vi "Autonomous Independent.vi"() -> ()   [LabVIEW 2017]
doc: "This VI is called when autonomous begins, and will automatically be terminated when autonomous ends. You can carry out timed or sensor driven robot movement independently without needing to return to the caller."
uses:
  Step Autonomous/TypeDefAuto.ctl
  Step Autonomous/TypeDefEnumSelection.ctl
  <vilib>/Rock Robotics/Network Tables/NT Read String.vi
  <vilib>/Rock Robotics/Network Tables/NT Write String.vi
  <vilib>/Rock Robotics/WPI/RobotDrive/WPI_RobotDriveArcadeDrive_Standard(NoSaturation).vi
  <vilib>/Rock Robotics/Network Tables/NT Write Numeric Array.vi
panel:
  out "directvi":string
  out "dashboard":string
  out "global":string
  out "Current Movement, for debugging":T1 {"Y Joystick Value" scale=1.0..-1.0; "X Joystick Value" scale=-1.0..1.0}
  in  "Array of robot movements":T2(array[cluster])=[{"X Joystick Value"=0.39393939393939403, "Y Joystick Value"=0.0, "Delay (sec)"=1.0, "Movement Name"="turn"}, {"X Joystick Value"=-0.3737373737373737, "Y Joystick Value"=0.0, "Delay (sec)"=1.0, "Movement Name"="turn back"}] {"Y Joystick Value" scale=1.0..-1.0; "X Joystick Value" scale=-1.0..1.0}
  # "Be sure to right-click and choose Data Operations>>Make Current Value default if you want to save the array values with the VI"
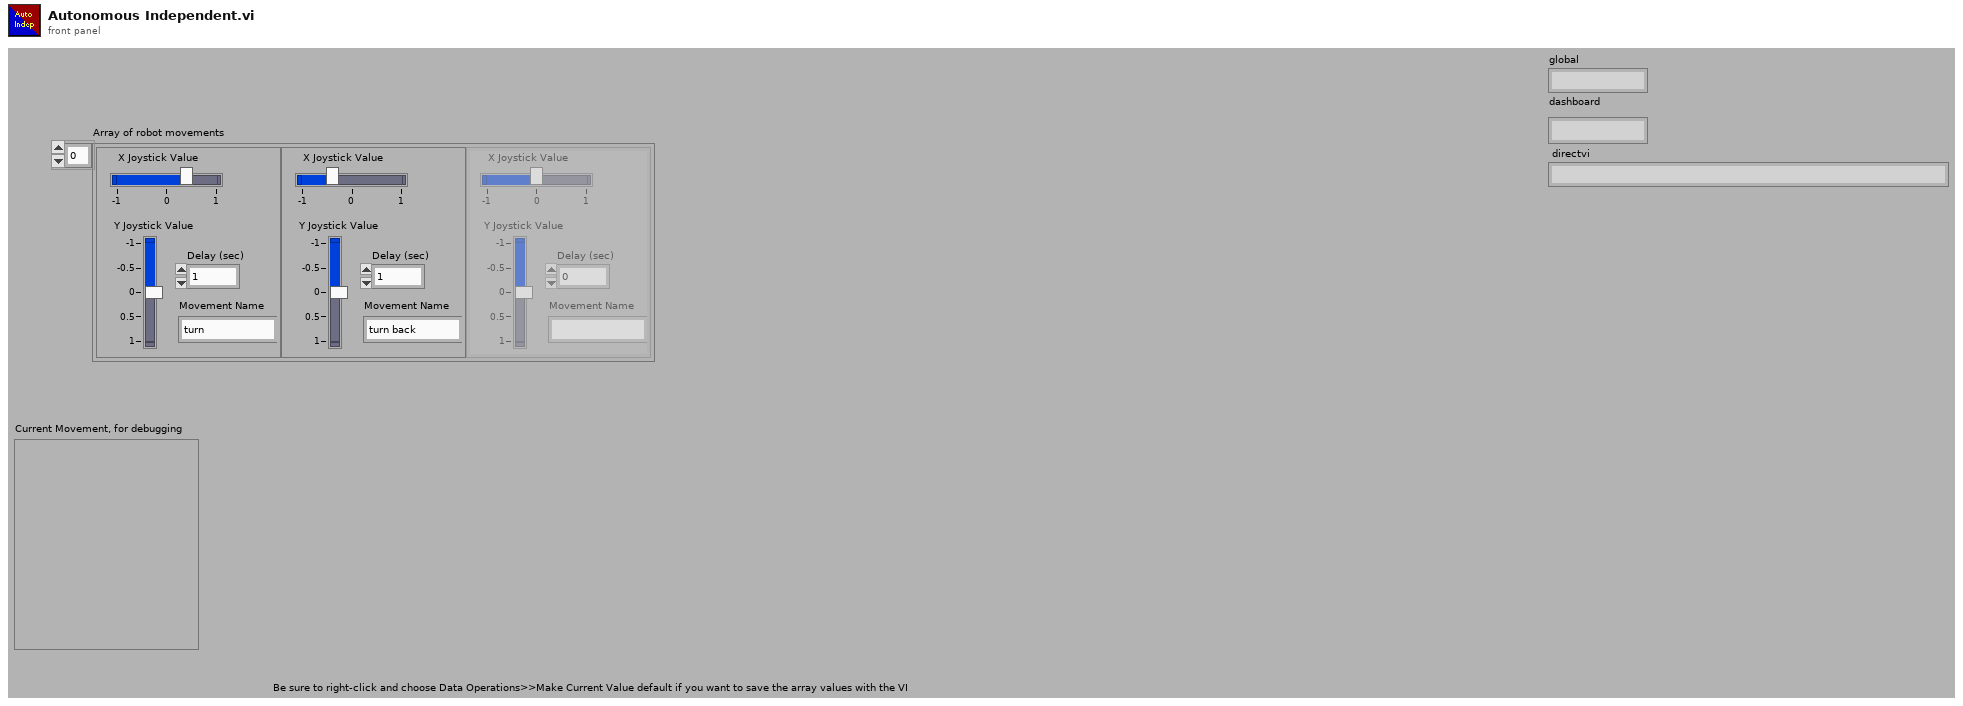
[diagram p1: front panel]
types:
  T1 = cluster{"X Joystick Value":dbl, "Y Joystick Value":dbl, "Delay (sec)":dbl, "Movement Name":string}
  T2 = cluster{"X Joystick Value":dbl, "Y Joystick Value":dbl, "Delay (sec)":dbl, "Movement Name":string}[]
  T3 = typedef "WPI_RobotDriveDevRef.ctl" = cluster{"DevStatus":errorcluster, "Motors[]":T4[], "Square Inputs":bool, "Max Output":dbl}
  T4 = typedef "WPI_MotorControlDeviceRef.ctl" = cluster{"DeviceStatus":errorcluster, "Type":T5, "PWM":cluster{"PWM Channel":T6, "DeadBand":T7}, "CAN":cluster{"Device Number":u8, "SetOutput VI Ref":variant, "GetOutput VI Ref":variant, "Enable VI Ref":variant, "Disable VI Ref":variant, "Data":variant}, "Invert":bool, "DIO PWM":cluster{"PWM \"Enable\" Channel":T6, "DIOChannel":T8, "PWM Rate":dbl}}
  T5 = typedef "WPI_MotorControlType.ctl" = enum16{"PWM", "CAN", "DIO PWM"}
  T6 = typedef "FPGA_DIOPWMChannel.ctl" = enum8{"PWM 0", "PWM 1", "PWM 2", "PWM 3", "PWM 4", "PWM 5", "PWM 6", "PWM 7", "PWM 8", "PWM 9", "PWM MXP 0", "PWM MXP 1", "PWM MXP 2", "PWM MXP 3", "PWM MXP 4", "PWM MXP 5", "PWM MXP 6", "PWM MXP 7", "PWM MXP 8", "PWM MXP 9", "Invalid"}
  T7 = typedef "WPI_PWMDeadband.ctl" = cluster{"Name":string, "maxPositivePwm":i32, "minPositivePwm":i32, "centerPwm":i32, "maxNegativePwm":i32, "minNegativePwm":i32, "angularRange":u16}
  T8 = typedef "FPGA_DIOChannel.ctl" = enum8{"DIO 0", "DIO 1", "DIO 2", "DIO 3", "DIO 4", "DIO 5", "DIO 6", "DIO 7", "DIO 8", "DIO 9", "DIO MXP 0", "DIO MXP 1", "DIO MXP 2", "DIO MXP 3", "DIO MXP 4", "DIO MXP 5", "DIO MXP 6", "DIO MXP 7", "DIO MXP 8", "DIO MXP 9", "DIO MXP 10", "DIO MXP 11", "DIO MXP 12", "DIO MXP 13", "DIO MXP 14", "DIO MXP 15", "SPI Port CS1", "SPI Port CS2", "SPI Port CS3", "SPI Port MISO", "SPI Port MOSI", "Invalid"}
  T9 = typedef "TypeDefAuto.ctl" = cluster{"Selection":T10, "Magnitude":dbl}
  T10 = typedef "TypeDefEnumSelection.ctl" = enum16{"Intake", "Drive", "Turn", "Lift", "Eject", "Wait", "RaiseDrop", "FastDrive", "VisionDrive", "TimedDrive"}
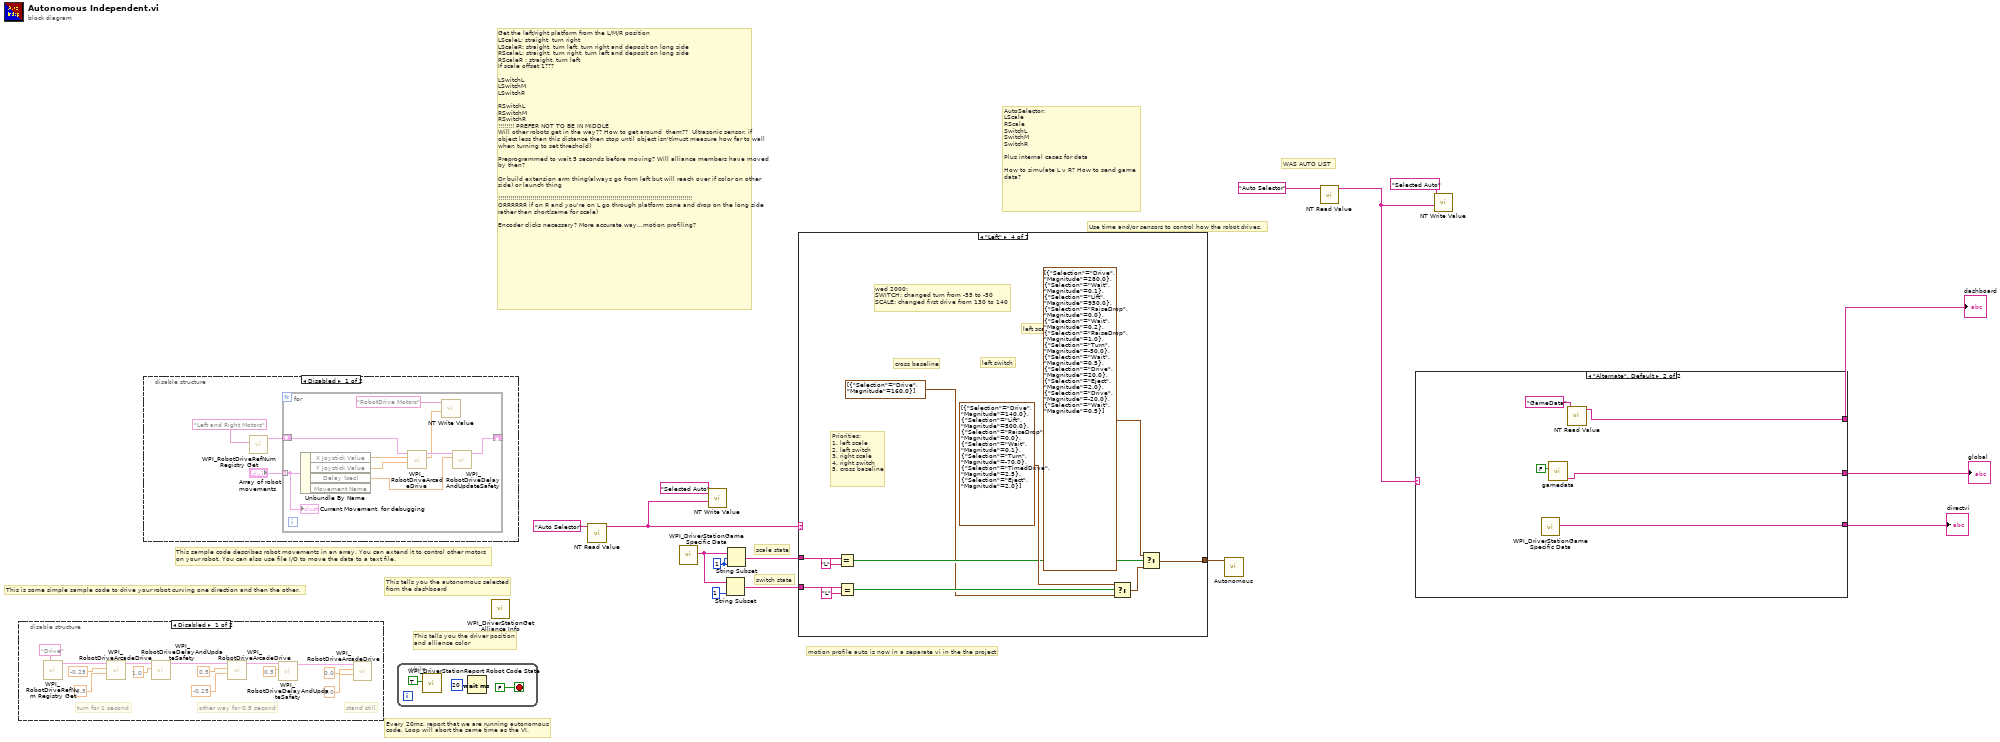
[diagram p0: block diagram]
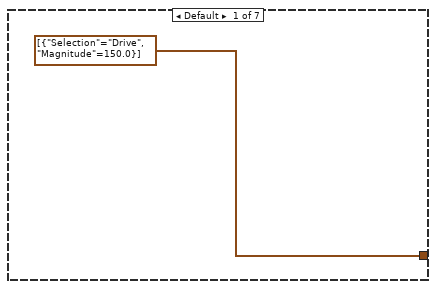
[diagram p2: hidden frame]
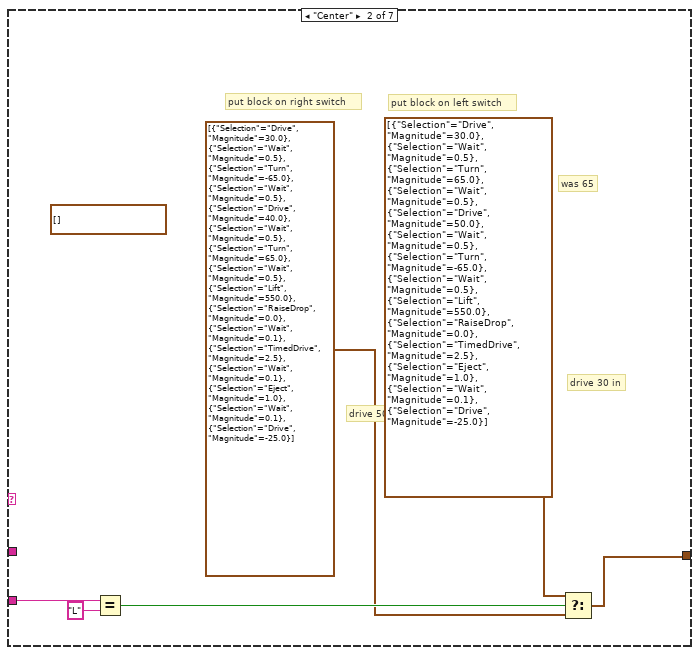
[diagram p3: hidden frame]
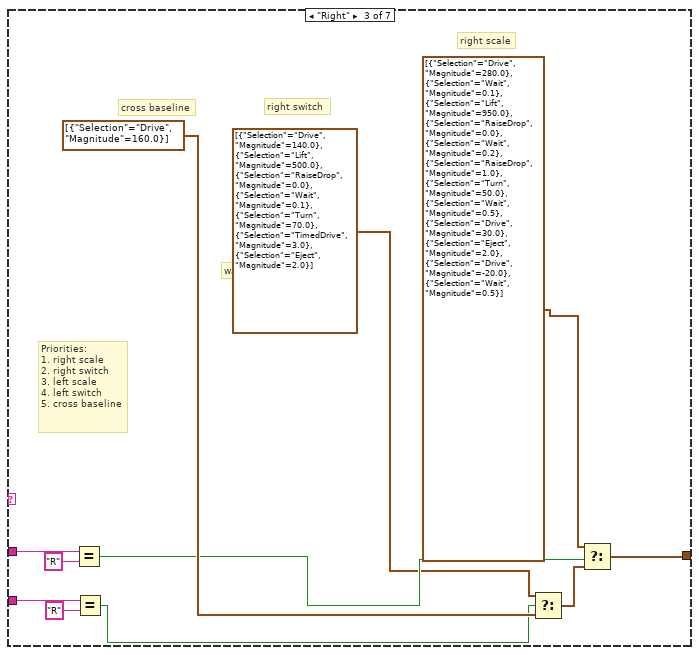
[diagram p4: hidden frame]
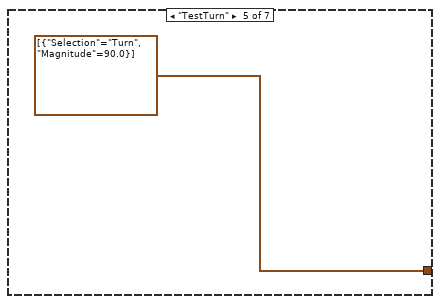
[diagram p5: hidden frame]
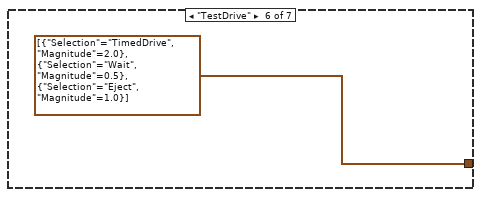
[diagram p6: hidden frame]
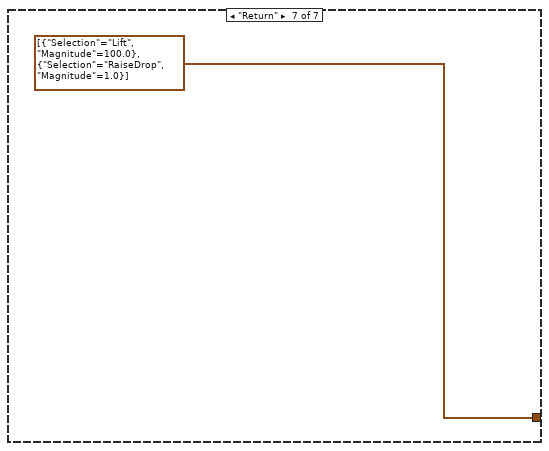
[diagram p7: hidden frame]
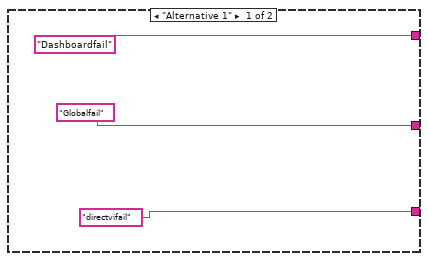
[diagram p8: hidden frame]
diagram:
  w2 = 1 ("length (rest)")
  # "motion profile auto is now in a separate vi in the the project"
  # "scale state"
  # "switch state"
  # "Use time and/or sensors to control how the robot drives."
  # "AutoSelector: \nLScale\nRScale\nSwitchL\nSwitchM\nSwitchR\n\nPlus internal cases for data\n\nHow to simulate L v R? How to send game data?"
  # "WAS AUTO LIST"
  # "This is some simple sample code to drive your robot curving one direction and then the other."
  # "This sample code describes robot movements in an array. You can extend it to control other motors\non your robot. You can also use file I/O to move the data to a text file."
  # "Get the left/right platform from the L/M/R position\nLScaleL: straight, turn right\nLScaleR: straight, turn left, turn right and deposit on long side\nRScaleL: straight, turn right, turn left and deposit on long side \nRScaleR : straight, turn left\nIf scale offset 1???\n\nLSwitchL\nLSwitchM\nLSwitchR\n\nRSwitchL\nRSwitchM\nRSwitchR\n!!!!!!!! PREFER NOT TO BE IN MIDDLE\nWill other robots get in the way?? How to get around  them??  Ultrasonic sensor, if object less than this distance then stop until object isn't(must measure how far to wall when turning to set threshold)\n\nPreprogrammed to wait 5 seconds before moving? Will alliance members have moved by then?\n\nOr build extension arm thing(always go from left but will reach over if color on other side) or launch thing\n\n!!!!!!!!!!!!!!!!!!!!!!!!!!!!!!!!!!!!!!!!!!!!!!!!!!!!!!!!!!!!!!!!!!!!!!!!!!!!!!!!!!!!!!!!!!!!!!!!!\nORRRRRR if on R and you're on L go through platform zone and drop on the long side rather than short(same for scale)  \n\nEncoder clicks necessary? More accurate way...motion profiling?"
  # "This tells you the autonomous selected\nfrom the dashboard"
  # "Every 20ms, report that we are running autonomous\ncode. Loop will abort the same time as the VI."
  # "This tells you the driver position\nand alliance color"
  n1 = disable-structure shown="Disabled" {
    frame Disabled {
      # "stand still"
      # "other way for 0.5 second"
      # "turn for 1 second"
      n2 = call <vilib>:"WPI_RobotDriveRefNum Registry Get.vi"("refnum name"="Drive") -> ("RobotDriveDevRef"=w25:T3)  [unwired: 1 in, 9 out]
      n3 = call-poly <vilib>:"WPI_RobotDriveArcadeDrive.vi"("Y axis value"=0.5 ("X axis value"), "X axis value"=-0.25, "RobotDriveDevRef"=w25) -> ("RobotDriveDevRef"=w29:T3)  [unwired: 1 in, 7 out]
      n4 = call <vilib>:"WPI_RobotDriveDelayAndUpdateSafety.vi"("Delay (s)"=1.0, "RobotDriveDevRef"=w29) -> ("RobotDriveDevRef 2"=w28:T3)  [unwired: 8 in, 1 out]
      n5 = call-poly <vilib>:"WPI_RobotDriveArcadeDrive.vi"("Y axis value"=-0.25 ("X axis value"), "X axis value"=0.5, "RobotDriveDevRef"=w28) -> ("RobotDriveDevRef"=w27:T3)  [unwired: 1 in, 7 out]
      n6 = call <vilib>:"WPI_RobotDriveDelayAndUpdateSafety.vi"("Delay (s)"=0.5, "RobotDriveDevRef"=w27) -> ("RobotDriveDevRef 2"=w26:T3)  [unwired: 8 in, 1 out]
      n7 = call-poly <vilib>:"WPI_RobotDriveArcadeDrive.vi"("Y axis value"=0.0 ("X axis value"), "X axis value"=0.0, "RobotDriveDevRef"=w26) -> ()  [unwired: 1 in, 8 out]
    }
    frame Enabled {
    }
  }
  n8 = disable-structure shown="Disabled" {
    frame Disabled {
      n9 = call <vilib>:"WPI_RobotDriveRefNum Registry Get.vi"("refnum name"="Left and Right Motors") -> ("RobotDriveDevRef"=w31:T3)  [unwired: 1 in, 9 out]
      n10 = for {
        shift-right: [w39] -> _
        shift-left: w31 -> [w40]
        tunnel: "Array of robot movements" -> [w35] mode=indexing
        n11 = Unbundle By Name(w35) -> ("X Joystick Value"=w38:dbl, "Y Joystick Value"=w37:dbl, "Delay (sec)"=w36:dbl)  [unwired: 1 out]
        n12 = call-poly <vilib>:"WPI_RobotDriveArcadeDrive.vi"("Y axis value"=w37, "X axis value"=w38, "RobotDriveDevRef"=w40) -> ("Motor Values"=w33:dbl[], "RobotDriveDevRef"=w41:T3)  [unwired: 1 in, 6 out]
        n13 = call-poly <vilib>:"NT Write Value.vi"("Numeric Array"=w33, "Name"="RobotDrive Motors") -> ()  [unwired: 9 in, 1 out]
        n14 = call <vilib>:"WPI_RobotDriveDelayAndUpdateSafety.vi"("Delay (s)"=w36, "RobotDriveDevRef"=w41) -> ("RobotDriveDevRef 2"=w39:T3)  [unwired: 8 in, 1 out]
        "Current Movement, for debugging" <- w35
      }
    }
    frame Enabled {
    }
  }
  n15 = while {
    stop <- FALSE stop-if-true
    n16 = call <vilib>:"WPI_DriverStationReport Robot Code State.vi"("Autonomous"=TRUE) -> ()  [unwired: 10 in, 1 out]
    n17 = Wait (ms)(milliseconds to wait=u32 20) -> ()  [unwired: 1 out]
  }
  n18 = call <vilib>:"WPI_DriverStationGet Alliance Info.vi"() -> ()  [unwired: 12 out]
  n19 = call-poly <vilib>:"NT Read Value.vi"("Name"="Auto Selector") -> ("String"=w8:string)  [unwired: 9 in, 1 out]
  n20 = call <vilib>:"WPI_DriverStationGame Specific Data.vi"() -> ("Game Specific Data"=w5:string)  [unwired: 11 in]
  n21 = call-poly <vilib>:"NT Write Value.vi"("String"=w8, "Name"="Selected Auto") -> ()  [unwired: 9 in, 1 out]
  n22 = String Subset(string=w5, length (rest)=1 ("length (rest)")) -> (substring=w3:string)  [unwired: 1 in]
  n23 = String Subset(string=w5, offset (0)=w2, length (rest)=w2) -> (substring=w6:string)
  n24 = case shown="\"Left\"" w8 {
    tunnel: w6 -> [_ _ w60 w71 _ _ _]
    tunnel: [T9[] [{"Selection"=enum."Drive", "Magnitude"=150.0}] ("Auto Steps") w50 w62 w73 T9[] [{"Selection"=enum."Turn", "Magnitude"=90.0}] ("Auto Steps") T9[] [{"Selection"=enum."TimedDrive", "Magnitude"=2.0}, {"Selection"=enum."Wait", "Magnitude"=0.5}, {"Selection"=enum."Eject", "Magnitude"=1.0}] ("Auto Steps") T9[] [{"Selection"=enum."Lift", "Magnitude"=100.0}, {"Selection"=enum."RaiseDrop", "Magnitude"=1.0}] ("Auto Steps")] -> w1
    tunnel: w3 -> [_ w48 w58 w69 _ _ _]
    frame Default {
    }
    frame "Center" {
      (unwired) T9[] [] ("Auto Steps")
      # "drive 50 in"
      # "drive 30 in"
      # "was 65"
      # "put block on right switch"
      # "put block on left switch"
      n25 = Equal?(x=w48, y="L") -> (x = y?=w49:bool)
      n26 = Select(t=T9[] [{"Selection"=enum."Drive", "Magnitude"=30.0}, {"Selection"=enum."Wait", "Magnitude"=0.5}, {"Selection"=enum."Turn", "Magnitude"=65.0}, {"Selection"=enum."Wait", "Magnitude"=0.5}, {"Selection"=enum."Drive", "Magnitude"=50.0}, {"Selection"=enum."Wait", "Magnitude"=0.5}, {"Selection"=enum."Turn", "Magnitude"=-65.0}, {"Selection"=enum."Wait", "Magnitude"=0.5}, {"Selection"=enum."Lift", "Magnitude"=550.0}, {"Selection"=enum."RaiseDrop", "Magnitude"=0.0}, {"Selection"=enum."TimedDrive", "Magnitude"=2.5}, {"Selection"=enum."Eject", "Magnitude"=1.0}, {"Selection"=enum."Wait", "Magnitude"=0.1}, {"Selection"=enum."Drive", "Magnitude"=-25.0}] ("Auto Steps"), s=w49, f=T9[] [{"Selection"=enum."Drive", "Magnitude"=30.0}, {"Selection"=enum."Wait", "Magnitude"=0.5}, {"Selection"=enum."Turn", "Magnitude"=-65.0}, {"Selection"=enum."Wait", "Magnitude"=0.5}, {"Selection"=enum."Drive", "Magnitude"=40.0}, {"Selection"=enum."Wait", "Magnitude"=0.5}, {"Selection"=enum."Turn", "Magnitude"=65.0}, {"Selection"=enum."Wait", "Magnitude"=0.5}, {"Selection"=enum."Lift", "Magnitude"=550.0}, {"Selection"=enum."RaiseDrop", "Magnitude"=0.0}, {"Selection"=enum."Wait", "Magnitude"=0.1}, {"Selection"=enum."TimedDrive", "Magnitude"=2.5}, {"Selection"=enum."Wait", "Magnitude"=0.1}, {"Selection"=enum."Eject", "Magnitude"=1.0}, {"Selection"=enum."Wait", "Magnitude"=0.1}, {"Selection"=enum."Drive", "Magnitude"=-25.0}] ("Auto Steps")) -> (s? t:f=w50:T9[])
    }
    frame "Right" {
      # "was 20"
      # "Priorities:\n1. right scale\n2. right switch\n3. left scale\n4. left switch\n5. cross baseline"
      # "right switch"
      # "right scale"
      # "cross baseline"
      n27 = Equal?(x=w60, y="R") -> (x = y?=w55:bool)
      n28 = Equal?(x=w58, y="R") -> (x = y?=w54:bool)
      n29 = Select(t=T9[] [{"Selection"=enum."Drive", "Magnitude"=140.0}, {"Selection"=enum."Lift", "Magnitude"=500.0}, {"Selection"=enum."RaiseDrop", "Magnitude"=0.0}, {"Selection"=enum."Wait", "Magnitude"=0.1}, {"Selection"=enum."Turn", "Magnitude"=70.0}, {"Selection"=enum."TimedDrive", "Magnitude"=3.0}, {"Selection"=enum."Eject", "Magnitude"=2.0}] ("Auto Steps"), s=w54, f=T9[] [{"Selection"=enum."Drive", "Magnitude"=160.0}] ("Auto Steps")) -> (s? t:f=w57:T9[])
      n30 = Select(t=T9[] [{"Selection"=enum."Drive", "Magnitude"=280.0}, {"Selection"=enum."Wait", "Magnitude"=0.1}, {"Selection"=enum."Lift", "Magnitude"=950.0}, {"Selection"=enum."RaiseDrop", "Magnitude"=0.0}, {"Selection"=enum."Wait", "Magnitude"=0.2}, {"Selection"=enum."RaiseDrop", "Magnitude"=1.0}, {"Selection"=enum."Turn", "Magnitude"=50.0}, {"Selection"=enum."Wait", "Magnitude"=0.5}, {"Selection"=enum."Drive", "Magnitude"=30.0}, {"Selection"=enum."Eject", "Magnitude"=2.0}, {"Selection"=enum."Drive", "Magnitude"=-20.0}, {"Selection"=enum."Wait", "Magnitude"=0.5}] ("Auto Steps"), s=w55, f=w57) -> (s? t:f=w62:T9[])
    }
    frame "Left" {
      # "wed 2000:\nSWITCH: changed turn from -55 to -50\nSCALE: changed first drive from 130 to 140"
      # "Priorities:\n1. left scale\n2. left switch\n3. right scale\n4. right switch\n5. cross baseline"
      # "left switch"
      # "left scale"
      # "cross baseline"
      n31 = Equal?(x=w71, y="L") -> (x = y?=w66:bool)
      n32 = Equal?(x=w69, y="L") -> (x = y?=w65:bool)
      n33 = Select(t=T9[] [{"Selection"=enum."Drive", "Magnitude"=140.0}, {"Selection"=enum."Lift", "Magnitude"=500.0}, {"Selection"=enum."RaiseDrop", "Magnitude"=0.0}, {"Selection"=enum."Wait", "Magnitude"=0.1}, {"Selection"=enum."Turn", "Magnitude"=-70.0}, {"Selection"=enum."TimedDrive", "Magnitude"=2.5}, {"Selection"=enum."Eject", "Magnitude"=2.0}] ("Auto Steps"), s=w65, f=T9[] [{"Selection"=enum."Drive", "Magnitude"=160.0}] ("Auto Steps")) -> (s? t:f=w68:T9[])
      n34 = Select(t=T9[] [{"Selection"=enum."Drive", "Magnitude"=280.0}, {"Selection"=enum."Wait", "Magnitude"=0.1}, {"Selection"=enum."Lift", "Magnitude"=950.0}, {"Selection"=enum."RaiseDrop", "Magnitude"=0.0}, {"Selection"=enum."Wait", "Magnitude"=0.2}, {"Selection"=enum."RaiseDrop", "Magnitude"=1.0}, {"Selection"=enum."Turn", "Magnitude"=-50.0}, {"Selection"=enum."Wait", "Magnitude"=0.5}, {"Selection"=enum."Drive", "Magnitude"=20.0}, {"Selection"=enum."Eject", "Magnitude"=2.0}, {"Selection"=enum."Drive", "Magnitude"=-20.0}, {"Selection"=enum."Wait", "Magnitude"=0.5}] ("Auto Steps"), s=w66, f=w68) -> (s? t:f=w73:T9[])
    }
    frame "TestTurn" {
    }
    frame "TestDrive" {
    }
    frame "Return" {
    }
  }
  n35 = call "Autonomous.vi"("Auto Step"=w1) -> ()  [unwired: 11 in]
  n36 = call-poly <vilib>:"NT Read Value.vi"("Name"="Auto Selector") -> ("String"=w12:string)  [unwired: 9 in, 1 out]
  n37 = case shown="\"Alternate\", Default" w12 {
    tunnel: ["Globalfail" w83] -> w11
    tunnel: ["Dashboardfail" w82] -> w10
    tunnel: ["directvifail" w80] -> w9
    frame "Alternative 1" {
    }
    frame "Alternate", Default {
      n38 = call <vilib>:"WPI_DriverStationGame Specific Data.vi"() -> ("Game Specific Data"=w80:string)  [unwired: 11 in]
      n39 = call "gamedata.vi"("set(T)/get(F) 2"=FALSE) -> ("s? t:f"=w83:string)  [unwired: 10 in]
      n40 = call-poly <vilib>:"NT Read Value.vi"("Name"="GameData") -> ("String"=w82:string)  [unwired: 9 in, 1 out]
    }
  }
  "global" <- w11
  "dashboard" <- w10
  "directvi" <- w9
  n41 = call-poly <vilib>:"NT Write Value.vi"("String"=w12, "Name"="Selected Auto") -> ()  [unwired: 9 in, 1 out]
